vi "Parse Port Setup.vi"(8 "error in":errorcluster, 11 "node in":refnum<k20>) -> (0 "error out":errorcluster, 2 "portSetup":T1, 3 "node out":refnum<k20>)   [LabVIEW 2020, in "AIM ARINC 664 Import.lvlib"]
uses:
  AIM ARINC 664 Import.lvlib
  _typedefs/port_setup.ctl
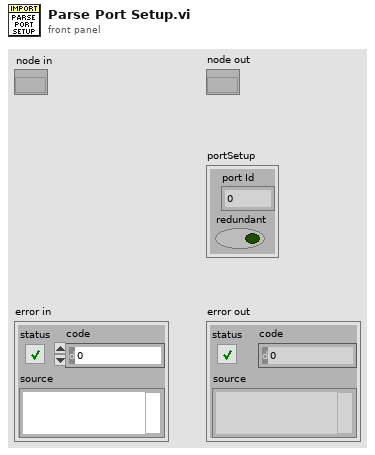
[diagram p1: front panel]
types:
  T1 = typedef "AIM ARINC 664 Import.lvlib/port_setup.ctl" = cluster{"port Id":u32, "redundant":bool}
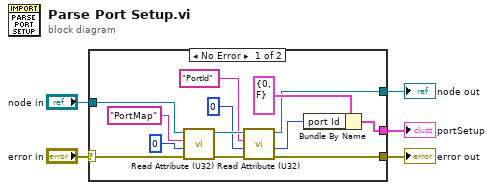
[diagram p0: block diagram]
diagram:
  n1 = case shown="No Error" "error in" {
    selector: "error in" -> [w11 w20]
    tunnel: "node in" -> [w16 w19]
    tunnel: [w9 w20] -> w4
    tunnel: [w18 _] -> w1
    tunnel: [w14 w19] -> w2
    frame No Error {
      n2 = call "Read Attribute (U32).vi"("error in"=w11, "default"=u32 0, "Attribute Name"="PortMap" ("Tag Name"), "node in"=w16) -> ("error out"=w10:errorcluster, "node out"=w15:refnum<k20>)  [unwired: 5 in, 1 out]
      n3 = call "Read Attribute (U32).vi"("error in"=w10, "default"=u32 0, "Attribute Name"="PortId" ("Tag Name"), "node in"=w15) -> ("error out"=w9:errorcluster, "value"=w8:u32, "node out"=w14:refnum<k20>)  [unwired: 5 in]
      n4 = Bundle By Name(cluster=T1 {"port Id"=0, "redundant"=FALSE} ("portSetup"), "port Id"=w8) -> (w18:T1)
    }
    frame Error {
    }
  }
  "error out" <- w4
  "node out" <- w2
  "portSetup" <- w1
